vi "Декодер.vi"(1 "Ответ Вх":u8[](array[numeric]) format="%02x") -> (0 "Ответ Вых":u8[](array[numeric]) format="%02x")   [LabVIEW 2010]
panel:
  out "SUB":bool
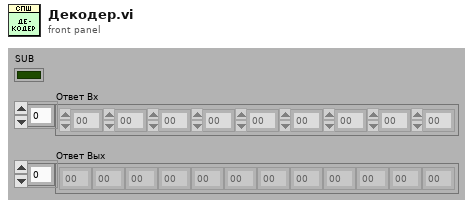
[diagram p1: front panel]
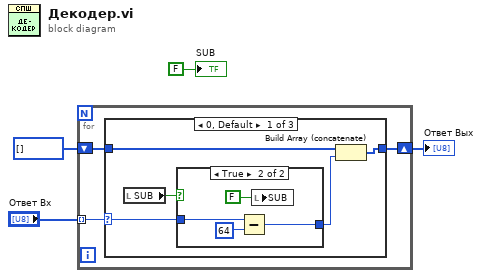
[diagram p0: block diagram]
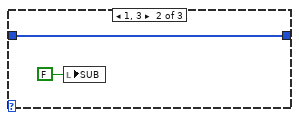
[diagram p3: hidden frame]
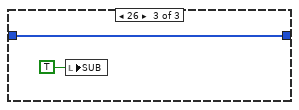
[diagram p4: hidden frame]
diagram:
  n1 = for {
    tunnel: "Ответ Вх" -> [w7] mode=indexing
    shift-right: [w5] -> w3
    shift-left: u8[] [] ("appended array") -> [w6]
    n2 = case shown="0, Default" w7 {
      selector: w7 -> [w9 _ _]
      tunnel: w6 -> [w12 w19 w20]
      tunnel: [w11 w19 w20] -> w5
      frame 0, Default {
        n3 = local read "SUB"() -> (w10:bool)
        n4 = case shown="True" w10 {
          tunnel: [w13 w15] -> w8
          tunnel: w9 -> [w13 w16]
          frame False {
          }
          frame True {
            n5 = Subtract(x=w16, y=u8 64 ("Numeric")) -> (x-y=w15:u8)
            n6 = local write "SUB"(FALSE ("SUB")) -> ()
          }
        }
        n7 = Build Array (concatenate)(w12, w8) -> (w11:u8[])
      }
      frame 1, 3 {
        n8 = local write "SUB"(FALSE ("SAB")) -> ()
      }
      frame 26 {
        n9 = local write "SUB"(TRUE ("SAB")) -> ()
      }
    }
  }
  "Ответ Вых" <- w3
  "SUB" <- FALSE ("SAB")
